vi "Begin.vi"() -> (0 "error out 5":errorcluster)   [LabVIEW 2013]
doc: "Called before other user functions, this VI is expected to open initial I/O refnums, load in file data, and do all program initialization. Notice that the <B>error out</B> terminal is simply used for data flow. Wiring it to other structures or subVIs ensures that this VI runs first."
uses:
  <vilib>/Rock Robotics/WPI/DriverStation/WPI_DriverStationRobotMode2.ctl
  <vilib>/Rock Robotics/WPI/SafetyOutput/WPI_SafetyOutputConfigMenu.ctl
  <vilib>/Rock Robotics/WPI/Joystick/WPI_JoystickDeviceEnum.ctl
  <vilib>/Rock Robotics/SystemInterfaces/DIO/FPGA_DIOPWMChannel.ctl
  <vilib>/Rock Robotics/WPI/Solenoid/WPI_SolenoidChannel.ctl
  <vilib>/Rock Robotics/SystemInterfaces/DIO/FPGA_DIORelayChannel.ctl
  <vilib>/Rock Robotics/SystemInterfaces/Typedef/FPGA_TypedefAnalogModule.ctl
  <vilib>/Rock Robotics/SystemInterfaces/AI/FPGA_AIChannel.ctl
  <vilib>/Rock Robotics/SystemInterfaces/Typedef/FPGA_TypedefDigitalModule.ctl
  <vilib>/Rock Robotics/SystemInterfaces/DIO/FPGA_DIOChannel.ctl
  <vilib>/Rock Robotics/WPI/Relay/WPI_RelayDirection.ctl
  <vilib>/Rock Robotics/SystemInterfaces/Typedef/FPGA_TypedefSolenoidModule.ctl
  Robot Global Data.vi
  <vilib>/Rock Robotics/WPI/Solenoid/WPI_SolenoidOpenDouble.vi
  <vilib>/Rock Robotics/WPI/MotorControl/WPI_MotorControlOpen Victor.vi
  <vilib>/Rock Robotics/WPI/RobotDrive/WPI_RobotDriveOpen4MotorWithVictor.vi
  <vilib>/Rock Robotics/WPI/Compressor/WPI_CompressorGetSetRefNum.vi
panel:
  out "error out 2":errorcluster
  out "error out 8":errorcluster
  out "error out 7":errorcluster
  out "error out 12":errorcluster
  out "error out 11":errorcluster
  out "error out 21":errorcluster
  out "error out 20":errorcluster
  out "error out 19":errorcluster
  out "error out 17":errorcluster
  out "error out 13":errorcluster
  out "error out 10":errorcluster
  out "error out 9":errorcluster
  out "error out 6":errorcluster
  out "error out":errorcluster
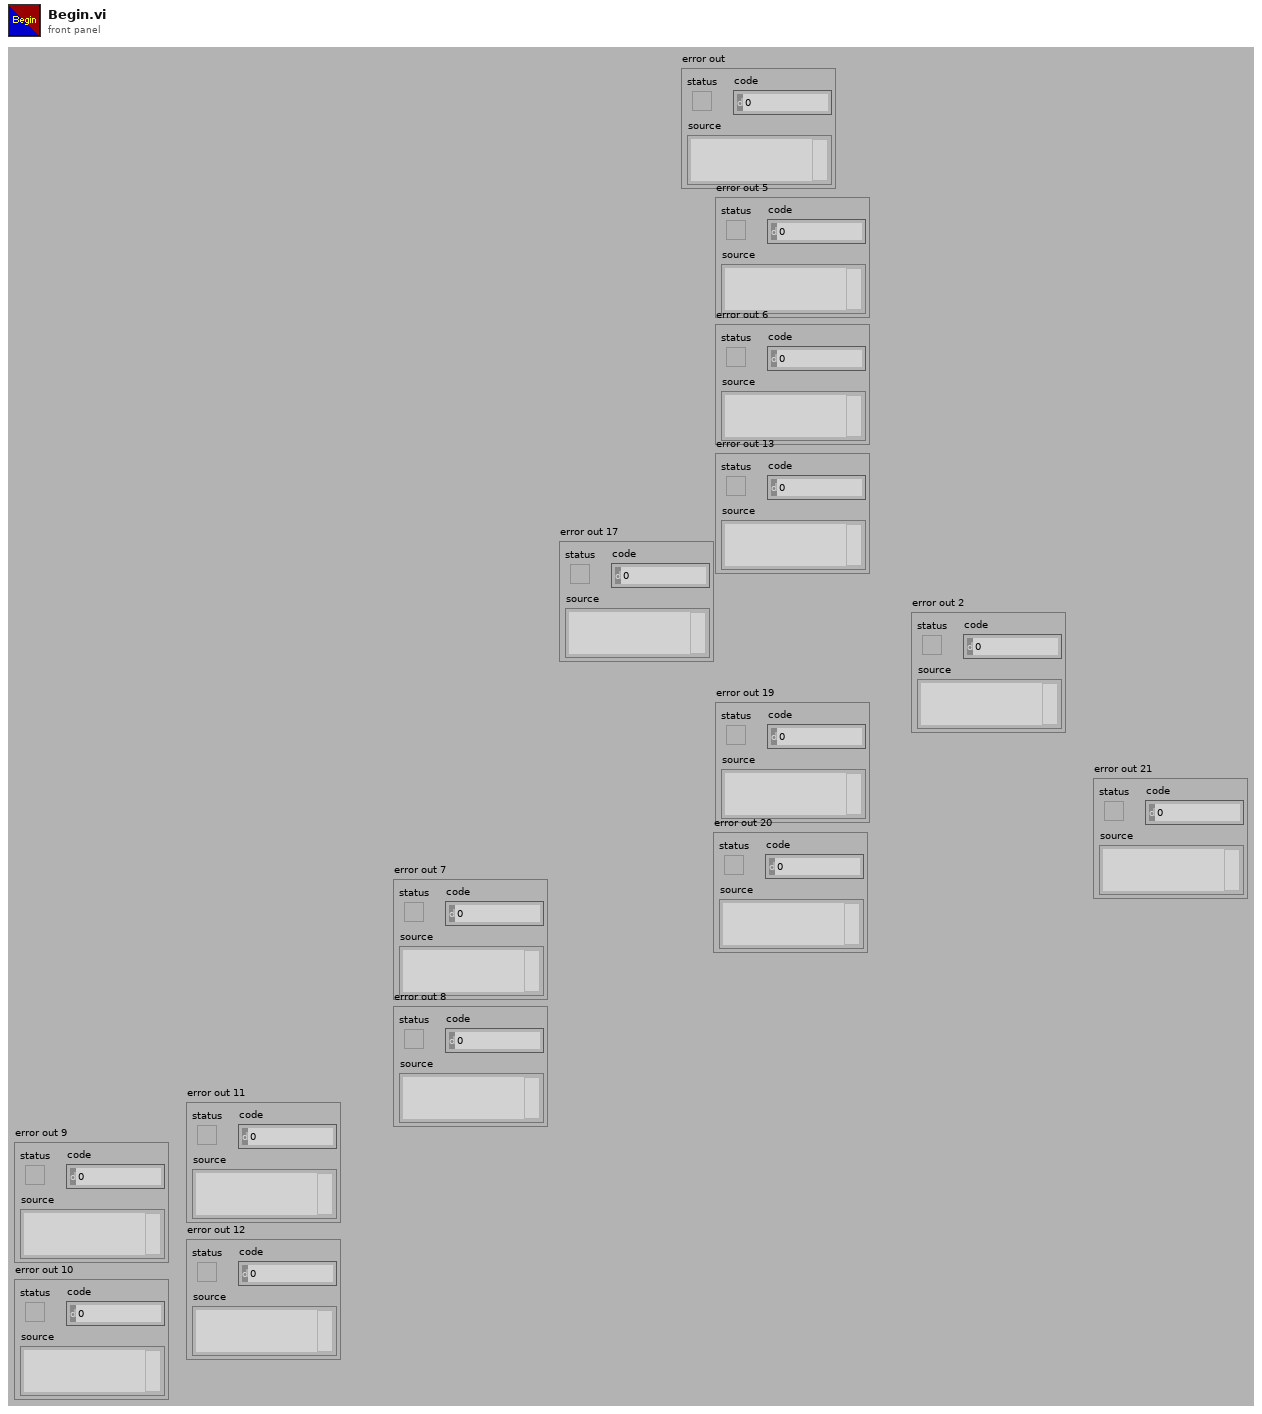
[diagram p1: front panel]
types:
  T1 = typedef "WPI_JoystickDeviceEnum.ctl" = enum16{"USB 1", "USB 2", "USB 3", "USB 4", "Kinect 1", "Kinect 2"}
  T2 = typedef "WPI_SafetyOutputConfigMenu.ctl" = enum16{"Enable", "Disable"}
  T3 = typedef "WPI_SolenoidChannel.ctl" = enum8{"Solenoid 1", "Solenoid 2", "Solenoid 3", "Solenoid 4", "Solenoid 5", "Solenoid 6", "Solenoid 7", "Solenoid 8", "Invalid"}
  T4 = typedef "FPGA_TypedefSolenoidModule.ctl" = enum16{"Solenoid Module 1", "Solenoid Module 2"}
  T5 = typedef "WPI_RelayDirection.ctl" = enum16{"Both directions", "Forward only", "Reverse only"}
  T6 = typedef "FPGA_DIORelayChannel.ctl" = enum8{"Relay 1", "Relay 2", "Relay 3", "Relay 4", "Relay 5", "Relay 6", "Relay 7", "Relay 8", "Invalid"}
  T7 = typedef "FPGA_TypedefDigitalModule.ctl" = enum16{"Digital Module 1", "Digital Module 2"}
  T8 = typedef "FPGA_DIOPWMChannel.ctl" = enum8{"PWM 1", "PWM 2", "PWM 3", "PWM 4", "PWM 5", "PWM 6", "PWM 7", "PWM 8", "PWM 9", "PWM 10", "Invalid"}
  T9 = typedef "FPGA_DIOChannel.ctl" = enum8{"DIO 1", "DIO 2", "DIO 3", "DIO 4", "DIO 5", "DIO 6", "DIO 7", "DIO 8", "DIO 9", "DIO 10", "DIO 11", "DIO 12", "DIO 13", "DIO 14", "Invalid"}
  T10 = typedef "FPGA_AIChannel.ctl" = enum8{"AI 1", "AI 2", "AI 3", "AI 4", "AI 5", "AI 6", "AI 7", "AI 8", "Invalid"}
  T11 = typedef "FPGA_TypedefAnalogModule.ctl" = enum16{"Analog Module 1", "Analog Module 2"}
  T12 = typedef "WPI_DriverStationRobotMode2.ctl" = enum16{"Autonomous Disabled", "Autonomous Enabled", "Teleop Disabled", "Teleop Enabled", "Timeout", "Finish", "Test Disabled", "Test Enabled"}
  T13 = typedef "WPI_RobotDriveDevRef.ctl" = cluster{"DevStatus":errorcluster, "Motors[]":T14[], "Square Inputs":bool, "Max Output":dbl, "Isochronous":bool}
  T14 = typedef "WPI_MotorControlDeviceRef.ctl" = cluster{"DeviceStatus":errorcluster, "Type":enum16{"PWM", "CAN"}, "PWM":cluster{"Digital Module":T7, "PWM Channel":T8, "DeadBand":T15}, "CAN":cluster{"Device Number":u8, "Control Mode":T16, "Semaphore":T17, "Max Vout":dbl}, "Invert":bool, "TransformRef":T18, "InvTransformRef":T18}
  T15 = typedef "WPI_PWMDeadband.ctl" = cluster{"Name":string, "maxPositivePwm":i32, "minPositivePwm":i32, "centerPwm":i32, "maxNegativePwm":i32, "minNegativePwm":i32, "angularRange":u16}
  T16 = typedef "WPI_CANJaguar_ControlMode.ctl" = enum8{"Percent VBus", "Current", "Speed", "Position", "Voltage"}
  T17 = typedef "Semaphore RefNum" = refnum<k1>
  T18 = typedef "WPI_PWMTransform_ConPane.ctl" = refnum<vi>
  T19 = typedef "WPI_RelayDevRef.ctl" = cluster{"DevStatus":errorcluster, "Relay Channel":T6, "Digital Module":T7, "Relay Direction":T5}
  T20 = typedef "WPI_CompressorDevRef.ctl" = cluster{"DevStatus":errorcluster, "DigitalInputDevRef":T21, "RelayDevRef":T19}
  T21 = typedef "WPI_DigitalInputDevRef.ctl" = cluster{"DevStatus":errorcluster, "DIO Channel":T9, "Digital Module":T7}
  T22 = typedef "WPI_SolenoidDevRef.ctl" = cluster{"DevStatus":errorcluster, "Solenoid Module":T4, "Forward Solenoid Channel":T3, "Reverse Solenoid Channel":T3}
  T23 = typedef "WPI_JoystickDevRef.ctl" = cluster{"Device":T1}
  T24 = typedef "WPI_AnalogChannelDevRef.ctl" = cluster{"DevStatus":errorcluster, "Analog Module":T11, "Analog Channel":T10}
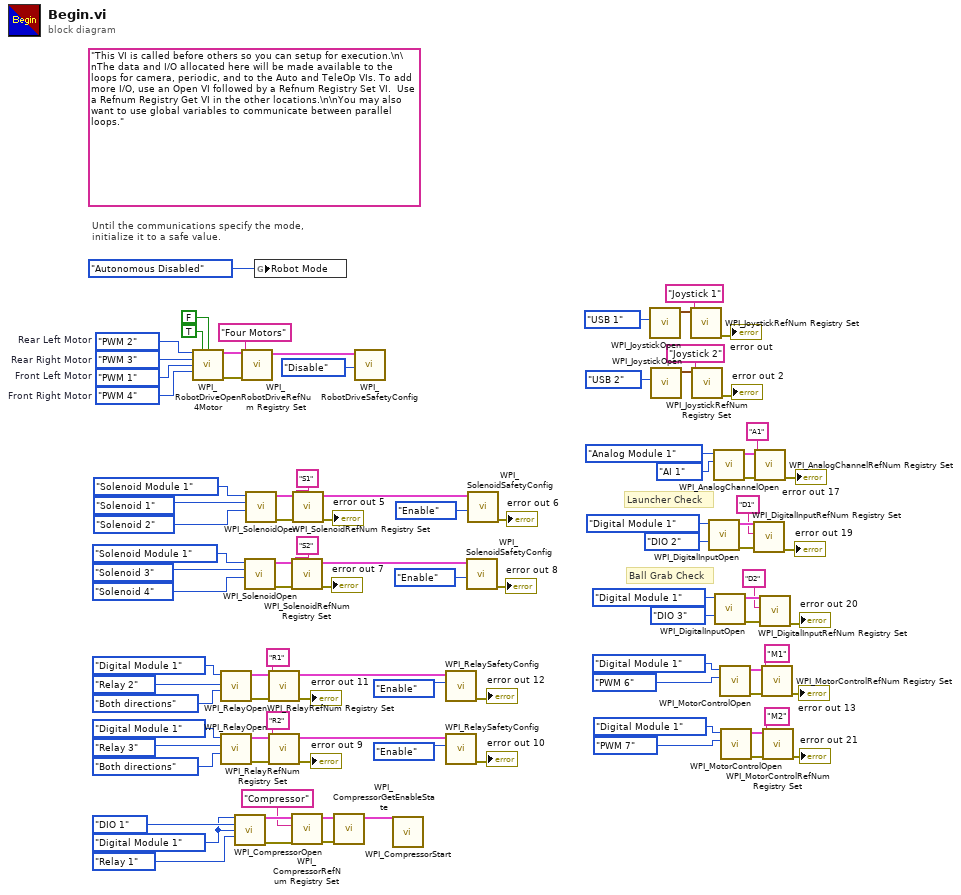
[diagram p0: block diagram]
diagram:
  w10 = TRUE ("Rear Right Motor Inverted")
  w9 = FALSE ("Rear Right Motor Inverted")
  w2 = FPGA_TypedefDigitalModule."Digital Module 1" ("Pressure Switch Digital Module (Module 1)")
  w88 = FPGA_DIOPWMChannel."PWM 4"  # Front Right Motor
  w89 = FPGA_DIOPWMChannel."PWM 1"  # Front Left Motor
  w90 = FPGA_DIOPWMChannel."PWM 3"  # Rear Right Motor
  w91 = FPGA_DIOPWMChannel."PWM 2"  # Rear Left Motor
  (unwired) "This VI is called before others so you can setup for execution.\n\nThe data and I/O allocated here will be made available to the loops for camera, periodic, and to the Auto and TeleOp VIs. To add more I/O, use an Open VI followed by a Refnum Registry Set VI.  Use a Refnum Registry Get VI in the other locations.\n\nYou may also want to use global variables to communicate between parallel loops."
  # "Ball Grab Check"
  # "Launcher Check"
  # "Until the communications specify the mode,\ninitialize it to a safe value."
  n1 = call-poly <vilib>:"WPI_RobotDriveOpen4Motor.vi"("Rear Left Motor"=w91, "Rear Left Motor Inverted"=w10, "Rear Right Motor Inverted"=w9, "Rear Right Motor"=w90, "Front Left Motor"=w89, "Front Right Motor"=w88, "Front Left Motor Inverted"=w10, "Front Right Motor Inverted"=w9) -> ("RobotDriveDevRef"=w8:T13, "error out"=w97:errorcluster)  [unwired: 6 in]
  n2 = call <vilib>:"WPI_RelayOpen.vi"("Relay Direction"=WPI_RelayDirection."Both directions", "Relay Channel"=FPGA_DIORelayChannel."Relay 2", "Digital Module (Module 1)"=FPGA_TypedefDigitalModule."Digital Module 1") -> ("error out"=w26:errorcluster, "RelayDevRef"=w28:T19)  [unwired: 7 in]
  n3 = call <vilib>:"WPI_RelayOpen.vi"("Relay Direction"=WPI_RelayDirection."Both directions", "Relay Channel"=FPGA_DIORelayChannel."Relay 3", "Digital Module (Module 1)"=FPGA_TypedefDigitalModule."Digital Module 1") -> ("error out"=w71:errorcluster, "RelayDevRef"=w73:T19)  [unwired: 7 in]
  n4 = call <vilib>:"WPI_CompressorOpen.vi"("Pressure Switch Digital Module (Module 1)"=w2, "Pressure Switch DIO Channel"=FPGA_DIOChannel."DIO 1", "Relay Digital Module (Module 1)"=w2, "Relay Channel"=FPGA_DIORelayChannel."Relay 1") -> ("CompressorDevRef"=w56:T20, "error out"=w53:errorcluster)  [unwired: 10 in]
  n5 = call <vilib>:"WPI_RobotDriveRefNum Registry Set.vi"("error in (no error)"=w97, "refnum name"="Four Motors", "RobotDriveDevRef"=w8) -> ("RobotDriveDevRef"=w96:T13)  [unwired: 8 out]
  n6 = call-poly <vilib>:"WPI_SolenoidOpen.vi"("Reverse Solenoid Channel"=WPI_SolenoidChannel."Solenoid 4", "Forward Solenoid Channel"=WPI_SolenoidChannel."Solenoid 3", "Solenoid Module (Module 1)"=FPGA_TypedefSolenoidModule."Solenoid Module 1") -> ("error out"=w16:errorcluster, "SolenoidDevRef"=w20:T22)  [unwired: 7 in]
  n7 = call-poly <vilib>:"WPI_SolenoidOpen.vi"("Reverse Solenoid Channel"=WPI_SolenoidChannel."Solenoid 2", "Forward Solenoid Channel"=WPI_SolenoidChannel."Solenoid 1", "Solenoid Module (Module 1)"=FPGA_TypedefSolenoidModule."Solenoid Module 1") -> ("error out"=w82:errorcluster, "SolenoidDevRef"=w86:T22)  [unwired: 7 in]
  n8 = global write "Robot Global Data.vi" "Robot Mode"(WPI_DriverStationRobotMode2."Autonomous Disabled" ("Robot Mode")) -> ()
  n9 = call <vilib>:"WPI_RelayRefNum Registry Set.vi"("error in (no error)"=w26, "refnum name"="R1", "RelayDevRef"=w28) -> ("error out"=→"error out 11":errorcluster, "RelayDevRef"=w25:T19)  [unwired: 7 in]
  n10 = call <vilib>:"WPI_RelayRefNum Registry Set.vi"("error in (no error)"=w71, "refnum name"="R2", "RelayDevRef"=w73) -> ("error out"=→"error out 9":errorcluster, "RelayDevRef"=w70:T19)  [unwired: 7 in]
  n11 = call <vilib>:"WPI_SolenoidRefNum Registry Set.vi"("error in (no error)"=w16, "refnum name"="S2", "SolenoidDevRef"=w20) -> ("error out"=→"error out 7":errorcluster, "SolenoidDevRef"=w15:T22)  [unwired: 7 in]
  n12 = call <vilib>:"WPI_CompressorRefNum Registry Set.vi"("error in (no error)"=w53, "refnum name"="Compressor", "CompressorDevRef"=w56) -> ("error out"=w51:errorcluster, "CompressorDevRef"=w50:T20)  [unwired: 7 in]
  n13 = call <vilib>:"WPI_SolenoidRefNum Registry Set.vi"("error in (no error)"=w82, "refnum name"="S1", "SolenoidDevRef"=w86) -> ("error out"=→"error out 5":errorcluster, "SolenoidDevRef"=w81:T22)  [unwired: 7 in]
  n14 = call <vilib>:"WPI_CompressorGetEnableState.vi"("error in (no error)"=w51, "CompressorDevRef"=w50) -> ("CompressorDevRef"=w1:T20)  [unwired: 6 in, 3 out]
  n15 = call <vilib>:"WPI_RobotDriveSafetyConfig.vi"("mode"=WPI_SafetyOutputConfigMenu."Disable", "RobotDriveDevRef"=w96) -> ()  [unwired: 8 in, 2 out]
  n16 = call <vilib>:"WPI_CompressorStart.vi"("CompressorDevRef"=w1) -> ()  [unwired: 9 in, 2 out]
  n17 = call <vilib>:"WPI_RelaySafetyConfig.vi"("mode"=WPI_SafetyOutputConfigMenu."Enable", "RelayDevRef"=w25) -> ("error out"=→"error out 12":errorcluster)  [unwired: 8 in, 1 out]
  n18 = call <vilib>:"WPI_RelaySafetyConfig.vi"("mode"=WPI_SafetyOutputConfigMenu."Enable", "RelayDevRef"=w70) -> ("error out"=→"error out 10":errorcluster)  [unwired: 8 in, 1 out]
  n19 = call <vilib>:"WPI_SolenoidSafetyConfig.vi"("mode"=WPI_SafetyOutputConfigMenu."Enable", "SolenoidDevRef"=w15) -> ("error out"=→"error out 8":errorcluster)  [unwired: 8 in, 1 out]
  n20 = call <vilib>:"WPI_SolenoidSafetyConfig.vi"("mode"=WPI_SafetyOutputConfigMenu."Enable", "SolenoidDevRef"=w81) -> ("error out"=→"error out 6":errorcluster)  [unwired: 8 in, 1 out]
  n21 = call <vilib>:"WPI_JoystickOpen.vi"("JoystickDevice"=WPI_JoystickDeviceEnum."USB 1") -> ("JoystickDevRef"=w93:T23)  [unwired: 10 in]
  n22 = call <vilib>:"WPI_JoystickOpen.vi"("JoystickDevice"=WPI_JoystickDeviceEnum."USB 2") -> ("JoystickDevRef"=w6:T23)  [unwired: 10 in]
  n23 = call <vilib>:"WPI_JoystickRefNum Registry Set.vi"("refnum name"="Joystick 1", "JoystickDevRef"=w93) -> ("error out"=→"error out":errorcluster)  [unwired: 8 in, 1 out]
  n24 = call <vilib>:"WPI_JoystickRefNum Registry Set.vi"("refnum name"="Joystick 2", "JoystickDevRef"=w6) -> ("error out"=→"error out 2":errorcluster)  [unwired: 8 in, 1 out]
  n25 = call <vilib>:"WPI_DigitalInputOpen.vi"("DIO Channel"=FPGA_DIOChannel."DIO 2", "Digital Module (Module 1)"=FPGA_TypedefDigitalModule."Digital Module 1") -> ("error out"=w49:errorcluster, "DigitalInputDevRef"=w48:T21)  [unwired: 8 in]
  n26 = call <vilib>:"WPI_AnalogChannelOpen.vi"("Analog Channel"=FPGA_AIChannel."AI 1", "Analog Module (Module 1)"=FPGA_TypedefAnalogModule."Analog Module 1") -> ("error out"=w61:errorcluster, "AIDeviceRef"=w60:T24)  [unwired: 8 in]
  n27 = call <vilib>:"WPI_DigitalInputOpen.vi"("DIO Channel"=FPGA_DIOChannel."DIO 3", "Digital Module (Module 1)"=FPGA_TypedefDigitalModule."Digital Module 1") -> ("error out"=w44:errorcluster, "DigitalInputDevRef"=w43:T21)  [unwired: 8 in]
  n28 = call-poly <vilib>:"WPI_MotorControlOpen.vi"("PWM Channel"=FPGA_DIOPWMChannel."PWM 6", "Digital Module (Module 1)"=FPGA_TypedefDigitalModule."Digital Module 1") -> ("error out"=w66:errorcluster, "MotorControlDeviceRef"=w65:T14)  [unwired: 8 in]
  n29 = call-poly <vilib>:"WPI_MotorControlOpen.vi"("PWM Channel"=FPGA_DIOPWMChannel."PWM 7", "Digital Module (Module 1)"=FPGA_TypedefDigitalModule."Digital Module 1") -> ("error out"=w36:errorcluster, "MotorControlDeviceRef"=w35:T14)  [unwired: 8 in]
  n30 = call <vilib>:"WPI_DigitalInputRefNum Registry Set.vi"("error in (no error)"=w49, "refnum name"="D1", "DigitalInputDevRef"=w48) -> ("error out"=→"error out 19":errorcluster)  [unwired: 7 in, 1 out]
  n31 = call <vilib>:"WPI_AnalogChannelRefNum Registry Set.vi"("error in (no error)"=w61, "refnum name"="A1", "AIDeviceRef"=w60) -> ("error out"=→"error out 17":errorcluster)  [unwired: 7 in, 1 out]
  n32 = call <vilib>:"WPI_DigitalInputRefNum Registry Set.vi"("error in (no error)"=w44, "refnum name"="D2", "DigitalInputDevRef"=w43) -> ("error out"=→"error out 20":errorcluster)  [unwired: 7 in, 1 out]
  n33 = call <vilib>:"WPI_MotorControlRefNum Registry Set.vi"("error in (no error)"=w66, "refnum name"="M1", "MotorControlDevRef"=w65) -> ("error out"=→"error out 13":errorcluster)  [unwired: 7 in, 1 out]
  n34 = call <vilib>:"WPI_MotorControlRefNum Registry Set.vi"("error in (no error)"=w36, "refnum name"="M2", "MotorControlDevRef"=w35) -> ("error out"=→"error out 21":errorcluster)  [unwired: 7 in, 1 out]
